vi "I2C Write.vi"() -> ()   [LabVIEW 2023, in "CTI-Visa-Scratchpad.lvlib"]
uses:
  CTI-Visa-Scratchpad.lvlib
  CTI-Visa/CTI-Visa.lvlib
panel:
  in  "Data":string
  in  "Address":u8 format="%.0x"
  in  "SDA GPIO":u8
  in  "SCL GPIO":u8
  in  "Baud":u32
  in  "Bus":u8
  out "error out":errorcluster
  in  "Port":refnum<visa-resource-name>="COM7"
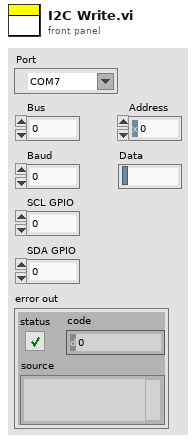
[diagram p1: front panel]
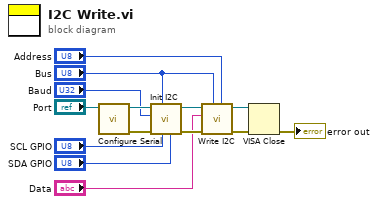
[diagram p0: block diagram]
diagram:
  n1 = call "Configure Serial.vi"("VISA resource name in"="Port") -> ("error out"=w13:errorcluster, "VISA resource name"=w12:refnum<visa-resource-name>)  [unwired: 9 in]
  n2 = call "Init I2C.vi"("SDA GPIO"="SDA GPIO", "SCL GPIO"="SCL GPIO", "Bus"="Bus", "error in (no error)"=w13, "Baud"="Baud", "VISA resource name in"=w12) -> ("error out"=w10:errorcluster, "VISA resource name"=w11:refnum<visa-resource-name>)  [unwired: 4 in]
  n3 = call "Write I2C.vi"("Address"="Address", "Bus"="Bus", "error in (no error)"=w10, "Data"="Data", "VISA resource name in"=w11) -> ("error out"=w9:errorcluster, "VISA resource name"=w8:refnum<visa-resource-name>)  [unwired: 5 in]
  n4 = VISA Close(VISA resource name=w8, error in (no error)=w9) -> (error out=→"error out":errorcluster)
